vi "toolkit-doc-generator-main.vi"(8 "error in":errorcluster, 9 "MTAdoc paths":path[](array[path]), 10 "VIs base path":path=path "/Macintosh HD/Users/oddoa/Work/LabVIEW/Vi-Documentation/TestViProject", 11 "report file destination":path=path "/Macintosh HD/Users/oddoa/Work/LabVIEW/Vi-Documentation/generated") -> (0 "error IO":errorcluster, 2 "vi paths":path[](array[path]), 3 "htmls generated":path[](array[path]))   [LabVIEW 2014]
uses:
  controls/state program.ctl
  controls/state-machine.ctl
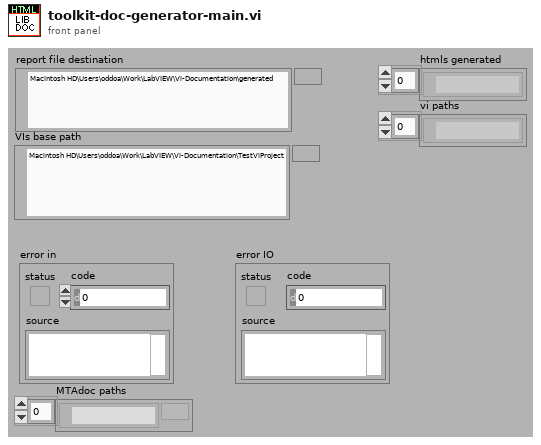
[diagram p1: front panel]
types:
  T1 = typedef "state program.ctl" = cluster{"State machine":T2, "HTML before":string, "HTML after":string}
  T2 = typedef "state-machine.ctl" = enum16{"add carridge return", "init", "Read-inputs", "edit generated file", "end", "Add front panel", "Add Block Diagram", "Add VI icon", "Add VI description", "Add VI hiearchy", "Add list of sub vis", "add custom html", "open report in browser", "Save report to file", "dispose report", "Add header text", "Create style .css", "add-red-box-header", "Delete Temp Files", "Remove-path-element", "add-revision-history", "add-icon-image-only"}
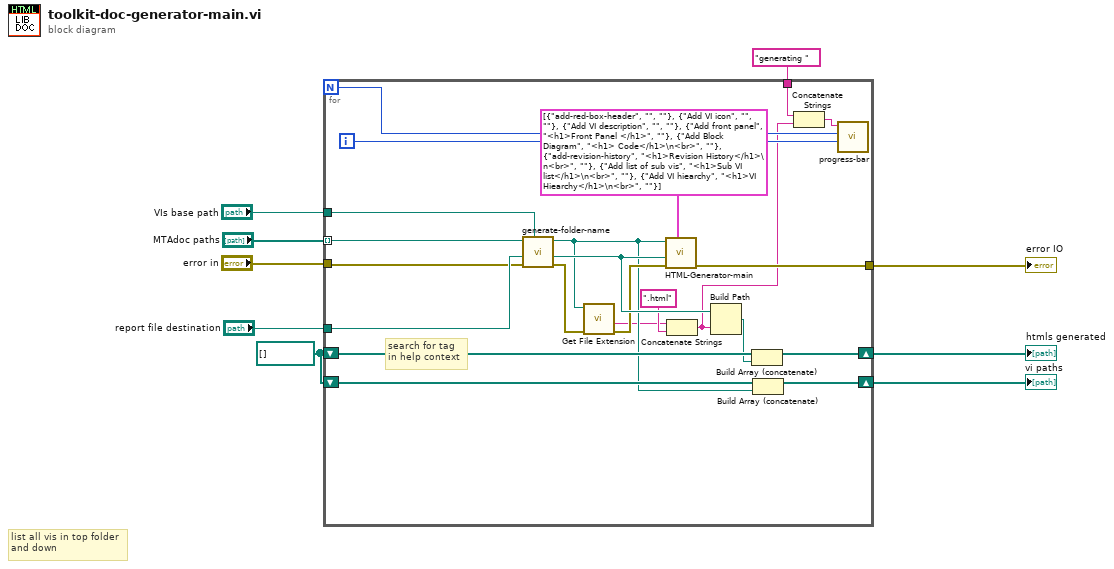
[diagram p0: block diagram]
diagram:
  w7 = path[] []
  # "list all vis in top folder\nand down"
  n1 = for {
    N -> [w24]
    tunnel: "report file destination" -> [w31]
    tunnel: "VIs base path" -> [w30]
    shift-right: [w28] -> w8
    shift-left: w7 -> [w29]
    shift-right: [w26] -> w6
    shift-left: w7 -> [w27]
    tunnel: "generating " -> [w23]
    tunnel: [w21] -> w4
    tunnel: "MTAdoc paths" -> [w20] mode=indexing
    tunnel: "error in" -> [w19]
    i -> [w25]
    # "search for tag\nin help context"
    n2 = call "generate-folder-name.vi"("vi path base"=w30, "error in"=w19, "report file destination base"=w31, "vi path"=w20) -> ("error out"=w15:errorcluster, "html destination"=w17:path, "vi path out"=w12:path)  [unwired: 5 out]
    n3 = call <vilib>:"Get File Extension.vi"("error in (no error)"=w15, "file"=w12) -> ("error out"=w14:errorcluster, "filename without extension"=w11:string)  [unwired: 8 out]
    n4 = call "HTML-Generator-main.vi"("tasks"=T1[] [{"State machine"=enum."add-red-box-header", "HTML before"="", "HTML after"=""}, {"State machine"=enum."Add VI icon", "HTML before"="", "HTML after"=""}, {"State machine"=enum."Add VI description", "HTML before"="", "HTML after"=""}, {"State machine"=enum."Add front panel", "HTML before"="<h1>Front Panel </h1>", "HTML after"=""}, {"State machine"=enum."Add Block Diagram", "HTML before"="<h1> Code</h1>\n<br>", "HTML after"=""}, {"State machine"=enum."add-revision-history", "HTML before"="<h1>Revision History</h1>\n<br>", "HTML after"=""}, {"State machine"=enum."Add list of sub vis", "HTML before"="<h1>Sub VI list</h1>\n<br>", "HTML after"=""}, {"State machine"=enum."Add VI hiearchy", "HTML before"="<h1>VI Hiearchy</h1>\n<br>", "HTML after"=""}], "error in"=w14, "report file destination"=w17, "VI path"=w12) -> ("error out"=w21:errorcluster)  [unwired: 1 in, 6 out]
    n5 = Concatenate Strings(w11, ".html" ("string")) -> (w10:string)
    n6 = Build Path(base path=w17, name or relative path=w10) -> (appended path=w13:path)
    n7 = Build Array (concatenate)(w29, w13) -> (w28:path[])
    n8 = Build Array (concatenate)(w27, w12) -> (w26:path[])
    n9 = Concatenate Strings(w23, w10) -> (w22:string)
    n10 = call "progress-bar.vi"("i++"=w25, "max"=w24, "state"=w22) -> ()  [unwired: 9 out]
  }
  "error IO" <- w4
  "htmls generated" <- w8
  "vi paths" <- w6
